vi "用户管理.vi"() -> (3 "字符串":string)   [LabVIEW 2016]
uses:
  <vilib>/Utility/file.llb/Read Delimited Spreadsheet (string).vi
  <vilib>/Utility/file.llb/Write Delimited Spreadsheet (string).vi
panel:
  out "布尔":bool
  in  "选中的工号":string
  in  "选中的姓名":string
  in  "修改用户":bool
  out "选中的行":i32
  in  "删除用户":bool
  in  "添加用户":bool
  in  "多列列表框":i32(listbox)
  in  "退出管理":bool
  # "用户管理界面"
  # "注：删除用户或修改用户前请先选中相应的行"
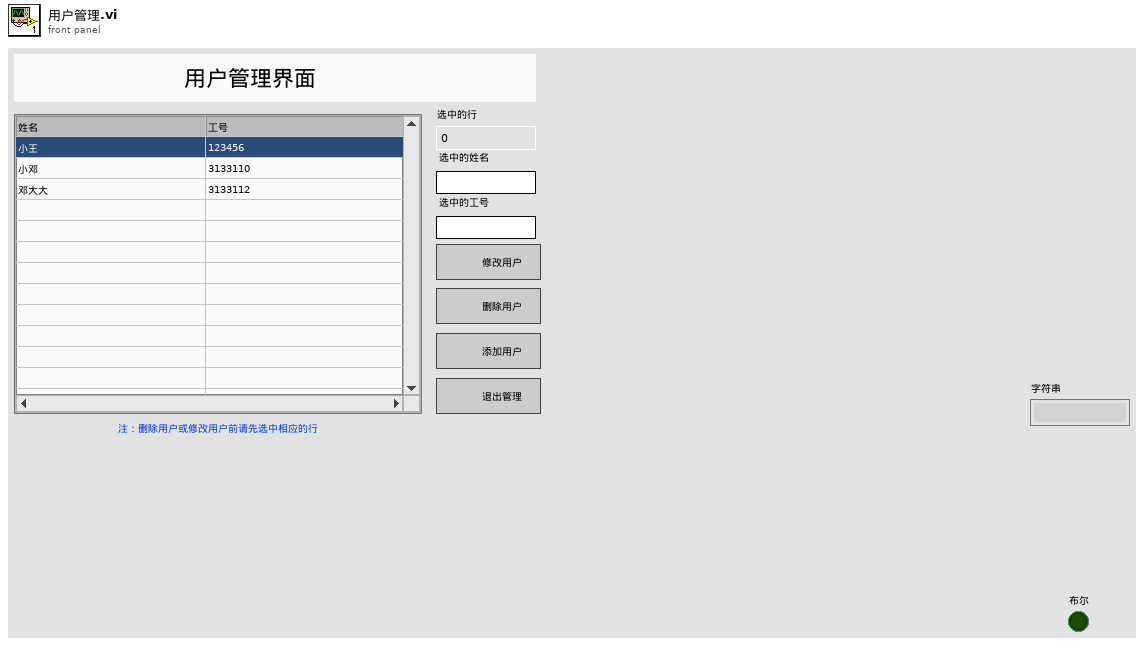
[diagram p1: front panel]
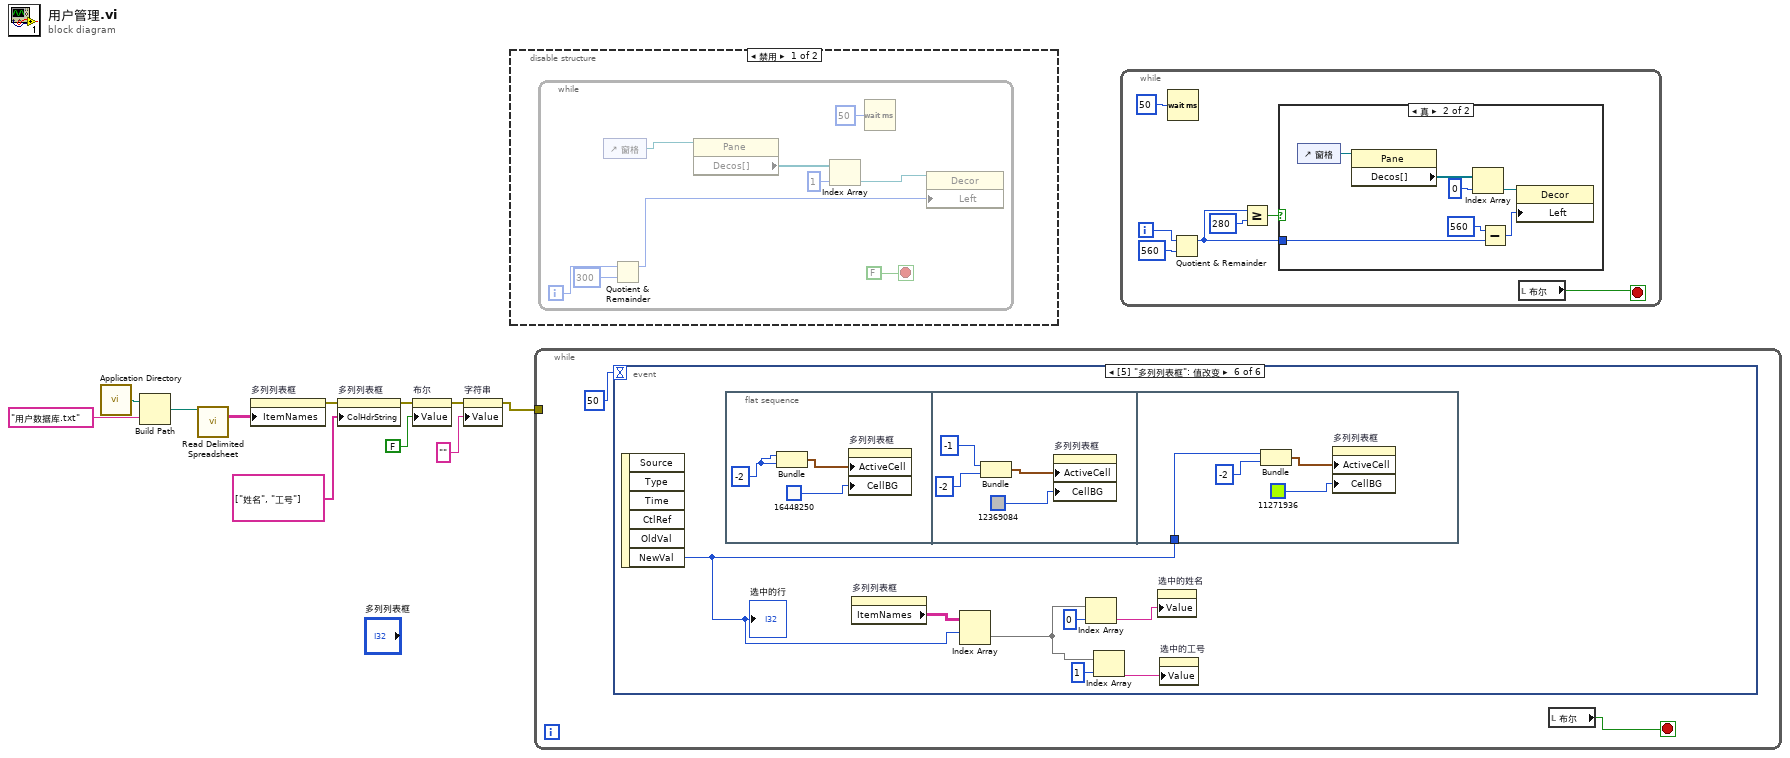
[diagram p0: block diagram]
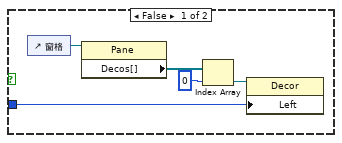
[diagram p3: hidden frame]
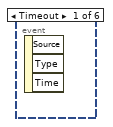
[diagram p4: hidden frame]
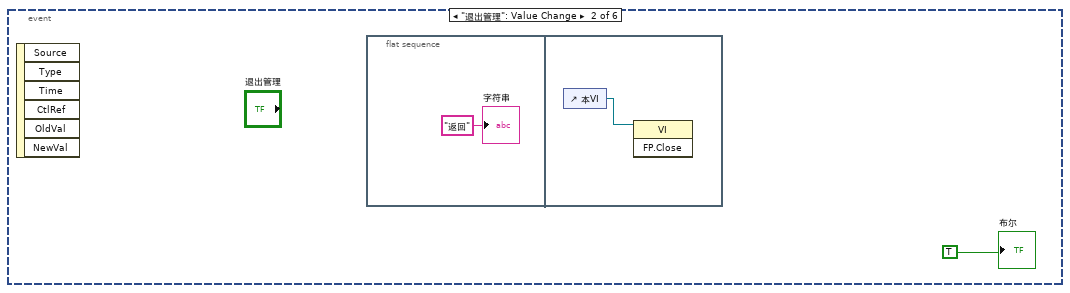
[diagram p5: hidden frame]
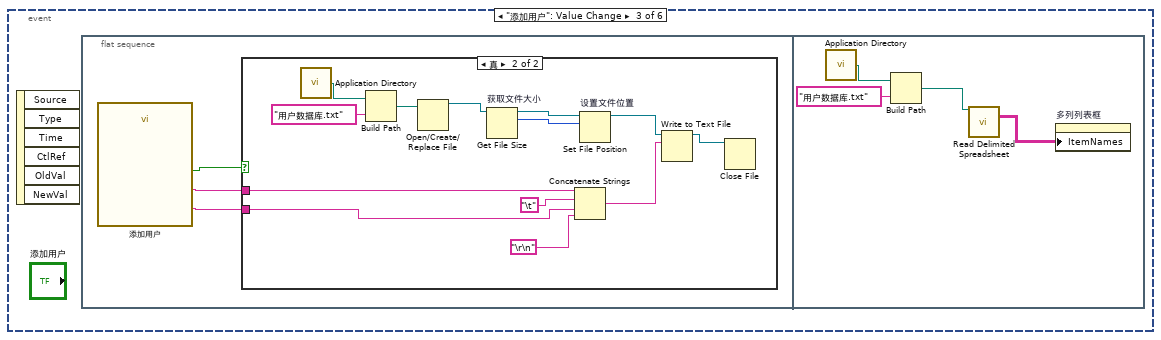
[diagram p6: hidden frame]
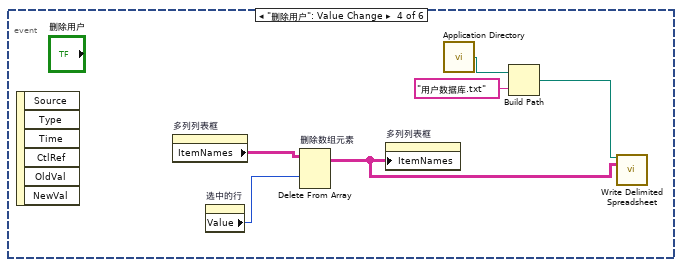
[diagram p8: hidden frame]
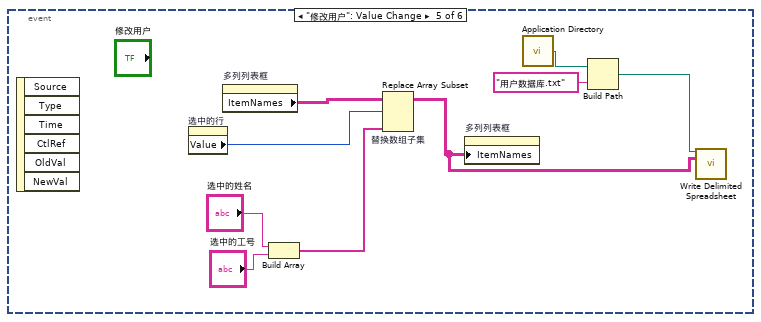
[diagram p9: hidden frame]
diagram:
  n1 = call <vilib>:"Application Directory.vi"() -> ("Application Directory"=w11:path)
  n2 = Build Path(base path=w11, name or relative path="用户数据库.txt" ("名称或相对路径")) -> (appended path=w9:path)
  n3 = call-poly <vilib>:"Read Delimited Spreadsheet.vi"("file path (dialog if empty)"=w9) -> ("all rows"=w8:string[][])  [unwired: 9 in, 5 out]
  n4 = property on="多列列表框" class="MCListbox (严格)"("ItemNames"=w8) -> (error out=w6:errorcluster)  [unwired: 2 in, 1 out]
  n5 = property on="多列列表框" class="MCListbox (严格)"(error in=w6, "ColHdrString"=string[] ["姓名", "工号"] ("列首字符串[]")) -> (error out=w4:errorcluster)  [unwired: 1 in, 1 out]
  n6 = property on="布尔" class="Bool (严格)"(error in=w4, "Value"=FALSE ("布尔")) -> (error out=w3:errorcluster)  [unwired: 1 in, 1 out]
  n7 = property on="字符串" class="Str"(error in=w3, "Value"="" ("字符串")) -> (error out=w2:errorcluster)  [unwired: 1 in, 1 out]
  n8 = disable-structure shown="禁用" {
    frame Disabled {
      n9 = while {
        i -> [w14]
        stop <- FALSE stop-if-true
        n10 = control-ref of="窗格"() -> (w20:refnum<vi>)
        n11 = Quotient & Remainder(x=w14, y=300) -> (x-y*floor(x/y)=w12:i32)  [unwired: 1 out]
        n12 = property class="Pane"(reference=w20) -> ("Decos[]"=w19:refnum<vi>[])  [unwired: 1 in, 2 out]
        n13 = Index Array(array=w19, index=1 ("索引")) -> (element=w17:refnum<vi>)
        n14 = Wait (ms)(milliseconds to wait=u32 50 ("等待时间（毫秒）")) -> ()  [unwired: 1 out]
        n15 = property class="Decor"(reference=w17, "Left"=w12) -> ()  [unwired: 1 in, 2 out]
      }
    }
    frame Enabled {
    }
  }
  n16 = while {
    tunnel: w2 -> [_]
    stop <- w21 stop-if-true
    n17 = event shown="[5] \"多列列表框\": 值改变" {
      selector: _ -> [_ _ _ _ _ _]
      dyn-events: _ -> [_ _ _ _ _ _]
      timeout: 50 -> [_ _ _ _ _ _]
      event Timeout {
        n18 = event-data() -> ()  [unwired: 1 in, 3 out]
      }
      event "退出管理": Value Change {
        n19 = event-data() -> ()  [unwired: 1 in, 6 out]
        n20 = flat-sequence {
          frame #0 {
            "字符串" <- "返回" ("字符串")
          }
          frame #1 {
            n21 = control-ref of="本VI"() -> (w25:refnum<vi>)
            n22 = invoke class="VI" method="FP.Close"(reference=w25) -> ()  [unwired: 2 in, 3 out]
          }
        }
        "布尔" <- TRUE
      }
      event "添加用户": Value Change {
        n23 = event-data() -> ()  [unwired: 1 in, 6 out]
        n24 = flat-sequence {
          frame #0 {
            n25 = call "添加用户"() -> ("密码"=w27:string, "用户名"=w28:string, "添加用户"=w26:bool)  [unwired: 16 in, 1 out]
            n26 = case shown="真" w26 {
              tunnel: w28 -> [_ w32]
              tunnel: w27 -> [_ w30]
              frame False {
              }
              frame True {
                n27 = call <vilib>:"Application Directory.vi"() -> ("Application Directory"=w40:path)
                n28 = Build Path(base path=w40, name or relative path="用户数据库.txt" ("名称或相对路径")) -> (appended path=w39:path)
                n29 = Open/Create/Replace File(file path (use dialog)=w39) -> (refnum out=w38:refnum<file>)  [unwired: 5 in, 2 out]
                n30 = Get File Size "获取文件大小"(file=w38) -> (refnum out=w37:refnum<file>, size (in bytes)=w36:i64)  [unwired: 1 in, 1 out]
                n31 = Concatenate Strings(w32, "\t", w30, "\r\n") -> (w33:string)
                n32 = Set File Position "设置文件位置"(offset (in bytes) (0)=w36, refnum=w37) -> (refnum out=w35:refnum<file>)  [unwired: 2 in, 1 out]
                n33 = Write to Text File(file (use dialog)=w35, text=w33) -> (refnum out=w34:refnum<file>)  [unwired: 2 in, 2 out]
                n34 = Close File(refnum=w34) -> ()  [unwired: 1 in, 2 out]
              }
            }
          }
          frame #1 {
            n35 = call <vilib>:"Application Directory.vi"() -> ("Application Directory"=w45:path)
            n36 = Build Path(base path=w45, name or relative path="用户数据库.txt" ("名称或相对路径")) -> (appended path=w43:path)
            n37 = call-poly <vilib>:"Read Delimited Spreadsheet.vi"("file path (dialog if empty)"=w43) -> ("all rows"=w42:string[][])  [unwired: 9 in, 5 out]
            n38 = property on="多列列表框" class="MCListbox (严格)"("ItemNames"=w42) -> ()  [unwired: 2 in, 2 out]
          }
        }
      }
      event "删除用户": Value Change {
        n39 = event-data() -> ()  [unwired: 1 in, 6 out]
        n40 = property on="多列列表框" class="MCListbox (严格)"() -> ("ItemNames"=w51:string[][])  [unwired: 2 in, 2 out]
        n41 = property on="选中的行" class="DigNum (严格)"() -> ("Value"=w50:i32)  [unwired: 2 in, 2 out]
        n42 = Delete From Array "删除数组元素"(array=w51, index (row)=w50) -> (array with subset deleted=w46:string[][])  [unwired: 2 in, 1 out]
        n43 = property on="多列列表框" class="MCListbox (严格)"("ItemNames"=w46) -> ()  [unwired: 2 in, 2 out]
        n44 = call <vilib>:"Application Directory.vi"() -> ("Application Directory"=w49:path)
        n45 = Build Path(base path=w49, name or relative path="用户数据库.txt" ("名称或相对路径")) -> (appended path=w47:path)
        n46 = call-poly <vilib>:"Write Delimited Spreadsheet.vi"("file path (dialog if empty)"=w47, "2D data"=w46) -> ()  [unwired: 12 in, 2 out]
      }
      event "修改用户": Value Change {
        n47 = event-data() -> ()  [unwired: 1 in, 6 out]
        n48 = property on="选中的行" class="DigNum (严格)"() -> ("Value"=w55:i32)  [unwired: 2 in, 2 out]
        n49 = property on="多列列表框" class="MCListbox (严格)"() -> ("ItemNames"=w57:string[][])  [unwired: 2 in, 2 out]
        n50 = Build Array("选中的姓名", "选中的工号") -> (w52:string[])
        n51 = Replace Array Subset "替换数组子集"(array=w57, new element=w52, index (row)=w55) -> (w56:string[][])  [unwired: 1 in]
        n52 = property on="多列列表框" class="MCListbox (严格)"("ItemNames"=w56) -> ()  [unwired: 2 in, 2 out]
        n53 = call <vilib>:"Application Directory.vi"() -> ("Application Directory"=w60:path)
        n54 = Build Path(base path=w60, name or relative path="用户数据库.txt" ("名称或相对路径")) -> (appended path=w58:path)
        n55 = call-poly <vilib>:"Write Delimited Spreadsheet.vi"("file path (dialog if empty)"=w58, "2D data"=w56) -> ()  [unwired: 12 in, 2 out]
      }
      event "多列列表框": Value Change {
        n56 = event-data() -> ("NewVal"=w66:i32)  [unwired: 1 in, 5 out]
        "选中的行" <- w66
        n57 = flat-sequence {
          tunnel: w66 -> [w78]
          frame #0 {
            w68 = -2
            n58 = Bundle(w68, w68) -> (w69:cluster{i32, i32})  [unwired: 1 in]
            n59 = property on="多列列表框" class="MCListbox (严格)"("ActiveCell"=w69, "CellBG"=u32 16448250) -> ()  [unwired: 2 in, 2 out]
          }
          frame #1 {
            n60 = Bundle(-1, -2) -> (w73:cluster{i32, i32})  [unwired: 1 in]
            n61 = property on="多列列表框" class="MCListbox (严格)"("ActiveCell"=w73, "CellBG"=u32 12369084) -> ()  [unwired: 2 in, 2 out]
          }
          frame #2 {
            n62 = Bundle("NewVal"=w78, -2) -> (w76:cluster{"NewVal":i32, i32})  [unwired: 1 in]
            n63 = property on="多列列表框" class="MCListbox (严格)"("ActiveCell"=w76, "CellBG"=u32 11271936) -> ()  [unwired: 2 in, 2 out]
          }
        }
        n64 = property on="多列列表框" class="MCListbox (严格)"() -> ("ItemNames"=w67:string[][])  [unwired: 2 in, 2 out]
        n65 = Index Array(array=w67, index (row)=w66) -> (element=w63:string[])  [unwired: 1 in]
        n66 = Index Array(array=w63, index=0 ("索引")) -> (element=w62:string)
        n67 = Index Array(array=w63, index=1 ("索引")) -> (element=w61:string)
        n68 = property on="选中的姓名" class="Str"("Value"=w62) -> ()  [unwired: 2 in, 2 out]
        n69 = property on="选中的工号" class="Str"("Value"=w61) -> ()  [unwired: 2 in, 2 out]
      }
    }
    n70 = local read "布尔"() -> (w21:bool)
  }
  n71 = while {
    i -> [w84]
    stop <- w79 stop-if-true
    n72 = Wait (ms)(milliseconds to wait=u32 50 ("等待时间（毫秒）")) -> ()  [unwired: 1 out]
    n73 = Quotient & Remainder(x=w84, y=560) -> (x-y*floor(x/y)=w82:i32)  [unwired: 1 out]
    n74 = Greater Or Equal?(x=w82, y=280) -> (x >= y?=w80:bool)
    n75 = case shown="真" w80 {
      tunnel: w82 -> [w86 w92]
      frame False {
        n76 = control-ref of="窗格"() -> (w90:refnum<vi>)
        n77 = property class="Pane"(reference=w90) -> ("Decos[]"=w89:refnum<vi>[])  [unwired: 1 in, 2 out]
        n78 = Index Array(array=w89, index=0 ("索引")) -> (element=w87:refnum<vi>)
        n79 = property class="Decor"(reference=w87, "Left"=w86) -> ()  [unwired: 1 in, 2 out]
      }
      frame True {
        n80 = control-ref of="窗格"() -> (w97:refnum<vi>)
        n81 = property class="Pane"(reference=w97) -> ("Decos[]"=w96:refnum<vi>[])  [unwired: 1 in, 2 out]
        n82 = Index Array(array=w96, index=0 ("索引")) -> (element=w94:refnum<vi>)
        n83 = Subtract(x=560 ("y"), y=w92) -> (x-y=w91:i32)
        n84 = property class="Decor"(reference=w94, "Left"=w91) -> ()  [unwired: 1 in, 2 out]
      }
    }
    n85 = local read "布尔"() -> (w79:bool)
  }
